vi "Get Type Priority.vi"(4 "Item Type":string) -> (1 "Priority":u32)   [LabVIEW 2020, in "AoC 2022.lvlib"]
uses:
  AoC 2022.lvlib
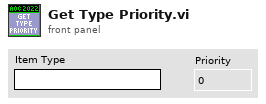
[diagram p1: front panel]
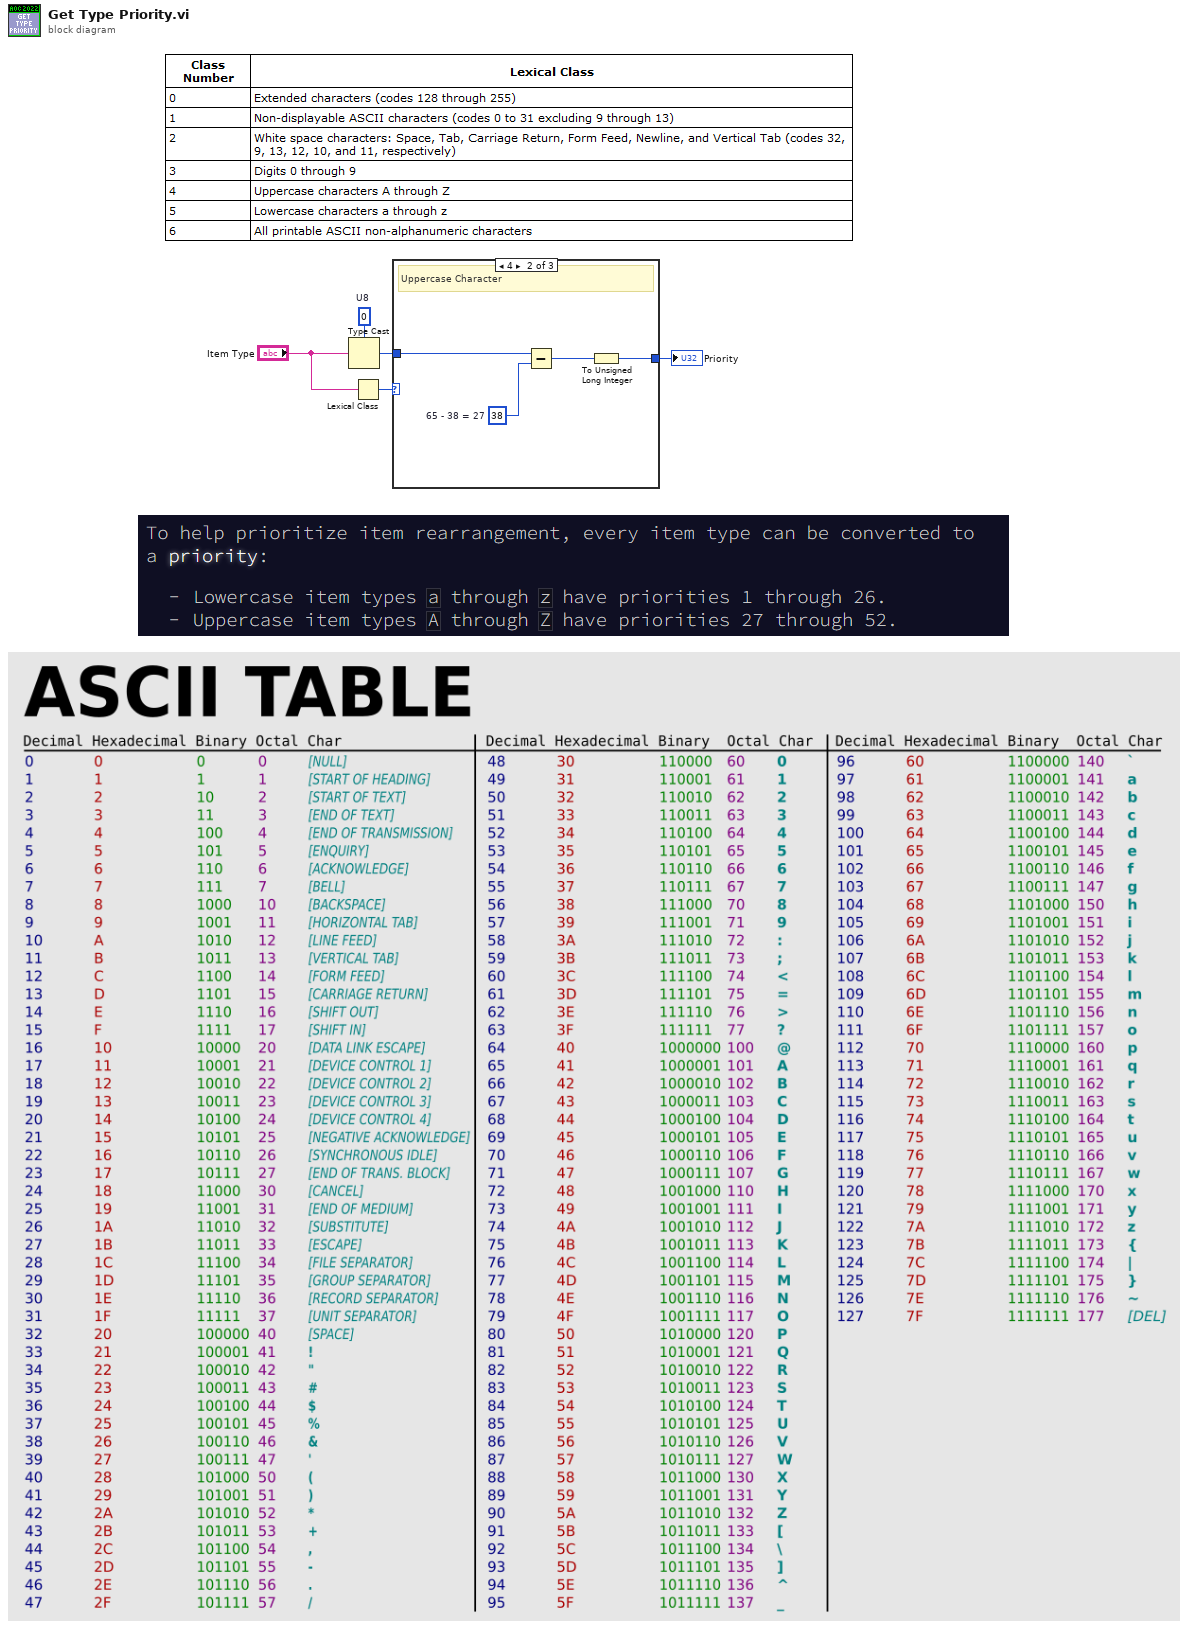
[diagram p0: block diagram]
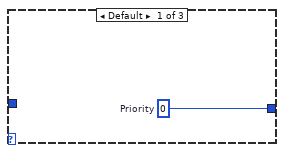
[diagram p2: hidden frame]
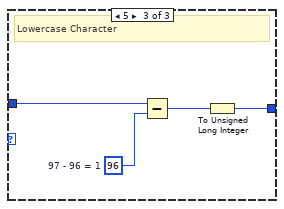
[diagram p3: hidden frame]
diagram:
  w3 = u8 0  # U8
  n1 = Type Cast(type=w3, x="Item Type") -> (*(type *) &x=w2:u8)
  n2 = Lexical Class(1:"Item Type") -> (0:w5:i16)
  n3 = case shown="4" w5 {
    tunnel: w2 -> [_ w10 w14]
    tunnel: [w6 w8 w12] -> w1
    frame Default {
      w6 = u32 0  # Priority
    }
    frame 4 {
      w7 = u8 38  # 65 - 38 = 27
      # "Uppercase Character"
      n4 = Subtract(x=w10, y=w7) -> (x-y=w9:u8)
      n5 = To Unsigned Long Integer(number=w9) -> (unsigned 32bit integer=w8:u32)
    }
    frame 5 {
      w11 = u8 96  # 97 - 96 = 1
      # "Lowercase Character"
      n6 = Subtract(x=w14, y=w11) -> (x-y=w13:u8)
      n7 = To Unsigned Long Integer(number=w13) -> (unsigned 32bit integer=w12:u32)
    }
  }
  "Priority" <- w1
